vi "typeDescriptor.vi"() -> (0 "defaultData":string, 1 "typeDescriptor":string)   [LabVIEW 2012, in "HGF_DeviceFSM.lvlib" / "HGF_TaskDFSM.lvclass"]
doc: "This VI returns the type descriptor and default data to be used by a PVPublisher."
uses:
  HGF_TaskDFSM.lvclass
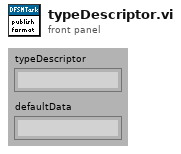
[diagram p1: front panel]
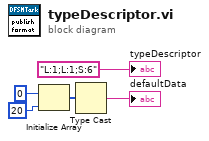
[diagram p0: block diagram]
diagram:
  n1 = Initialize Array(u8 0, 20 ("dimension size")) -> (w4:u8[])
  n2 = Type Cast(x=w4) -> (*(type *) &x=→"defaultData":string)  [unwired: 1 out]
  "typeDescriptor" <- "L:1;L:1;S:6" ("typeDescriptor")
